vi "Logging Message Loop.vi"(8 "error in (no error)":errorcluster, 10 "Data Queue":refnum<queue>, 11 "Message Queues":T1) -> (0 "error out":errorcluster)   [LabVIEW 2019, in "Logging.lvlib"]
doc: "The message loop subVI to handle messages pertaining to logging data."
uses:
  Logging.lvlib
  support/Message Queue/All Message Queues.ctl
  support/Message Queue/Message Cluster.ctl
  Logging Configuration.ctl
  support/Message Queue/Message Queue.lvlib
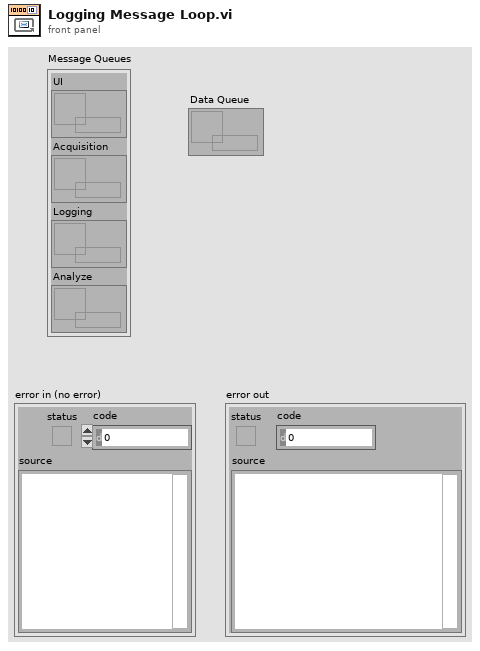
[diagram p1: front panel]
types:
  T1 = typedef "Message Queue.lvlib/All Message Queues.ctl" = cluster{"UI":refnum<queue>, "Acquisition":refnum<queue>, "Logging":refnum<queue>, "Analyze":refnum<queue>}
  T2 = typedef "Logging.lvlib/Logging Configuration.ctl" = cluster{"Log File Base Path":path, "Data Log Refnum":refnum<k1>}
  T3 = cluster{"Temperature Array":dbl[], "Average Range":dbl}
  T4 = enum16{"open", "replace", "create", "open or create", "replace or create", "replace or create with confirmation"}
  T5 = cluster{"Temperature Array":dbl[], "Average Range":dbl}[]
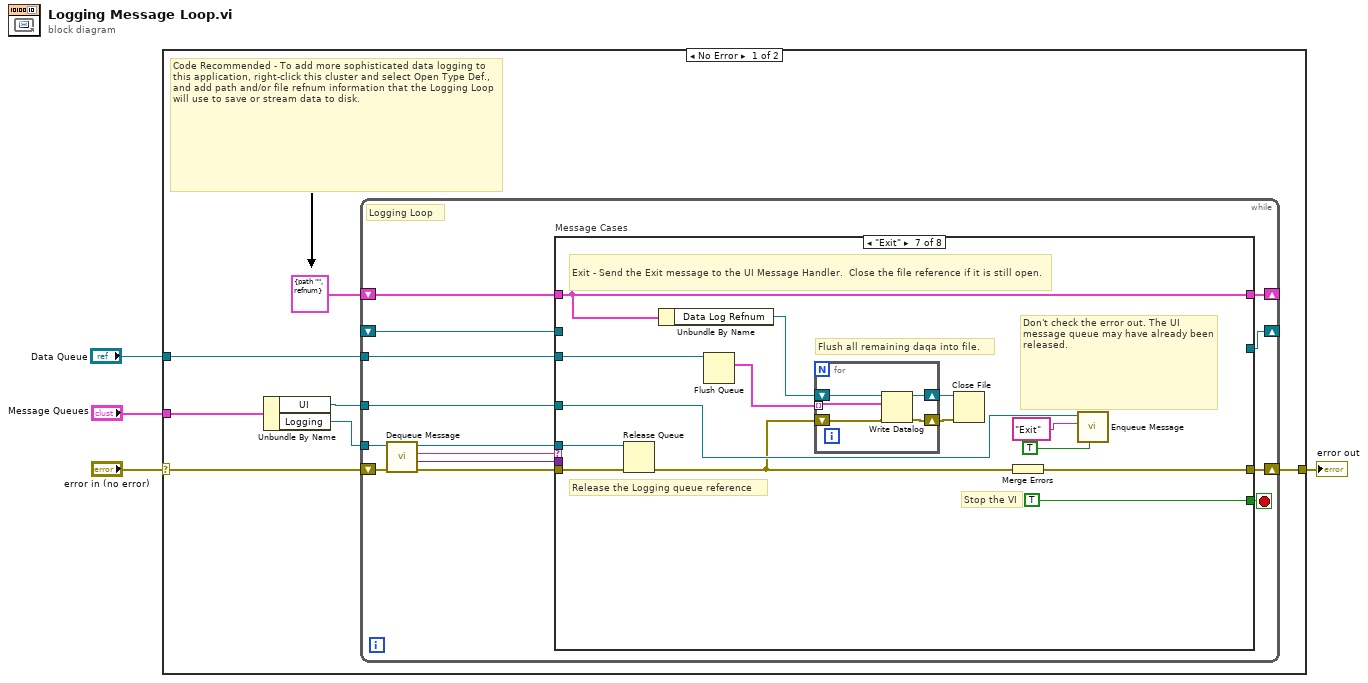
[diagram p0: block diagram]
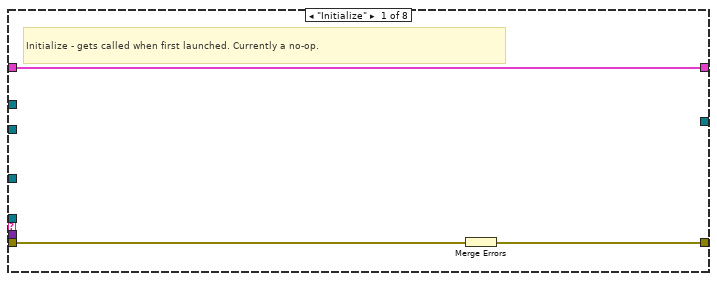
[diagram p2: hidden frame]
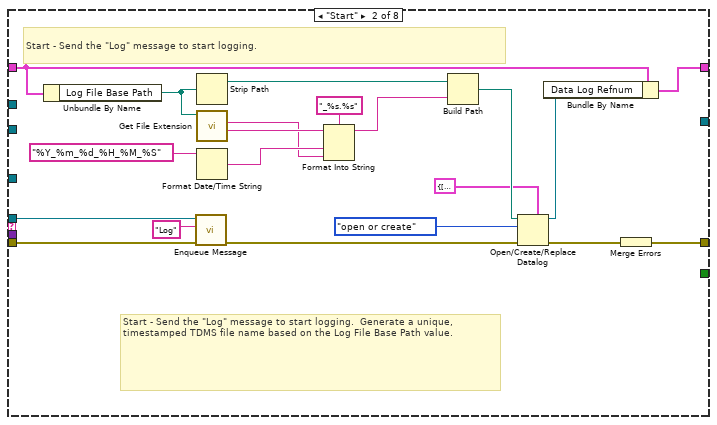
[diagram p3: hidden frame]
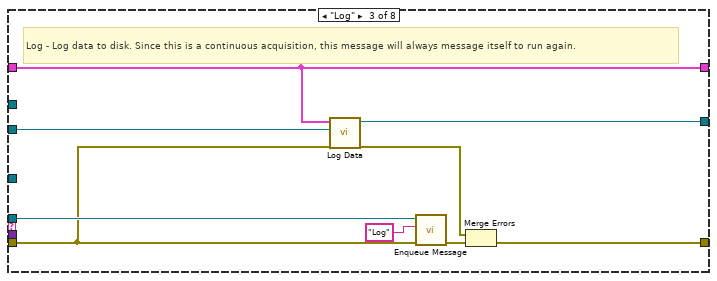
[diagram p4: hidden frame]
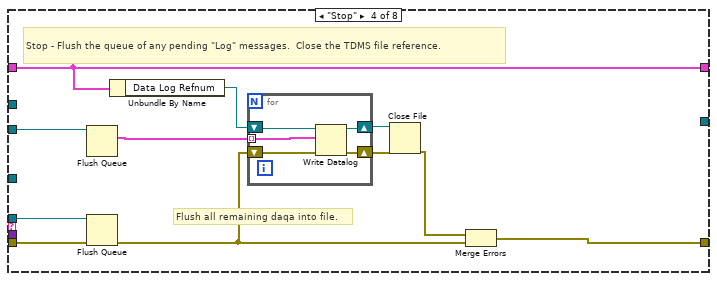
[diagram p5: hidden frame]
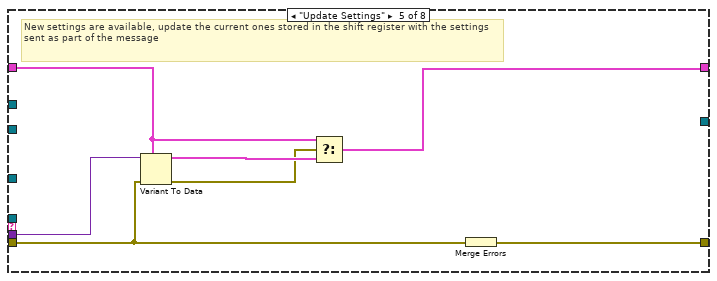
[diagram p6: hidden frame]
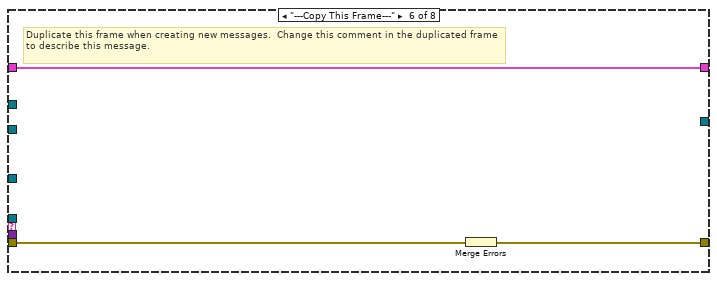
[diagram p7: hidden frame]
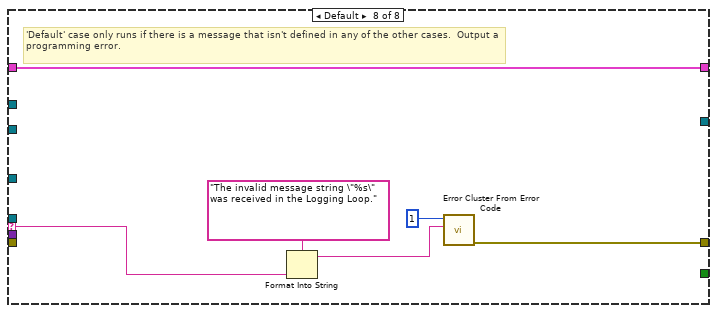
[diagram p8: hidden frame]
diagram:
  n1 = case shown="No Error" "error in (no error)" {
    selector: "error in (no error)" -> [w8 w109]
    tunnel: "Message Queues" -> [w11 _]
    tunnel: [w9 w109] -> w3
    tunnel: "Data Queue" -> [w7 _]
    frame No Error {
      # "Code Recommended - To add more sophisticated data logging to this application, right-click this cluster and select Open Type Def., and add path and/or file refnum information that the Logging Loop will use to save or stream data to disk."
      n2 = Unbundle By Name(w11) -> ("UI"=w6:refnum<queue>, "Logging"=w10:refnum<queue>)
      n3 = while {
        tunnel: w10 -> [w18]
        shift-right: [w24] -> w9
        shift-left: w8 -> [w23]
        tunnel: w6 -> [w17]
        tunnel: w7 -> [w16]
        shift-right: [w14] -> _
        shift-left: T2 {"Log File Base Path"=path "", "Data Log Refnum"=refnum} ("Logging Configuration") -> [w15]
        shift-right: [w13] -> _
        shift-left: _ -> [w12]
        stop <- w25 stop-if-true
        # "Logging Loop"
        n4 = call "Dequeue Message.vi"("error in (no error)"=w23, "Message Queue"=w18) -> ("error out"=w22:errorcluster, "Message Data"=w20:variant, "Message"=w21:string, "dup Message Queue"=w19:refnum<queue>)  [unwired: 6 in]
        n5 = case "Message Cases" shown="\"Exit\"" w21 {
          selector: w21 -> [_ _ _ _ _ _ _ w106]
          tunnel: w19 -> [_ w47 w55 w66 _ _ w91 _]
          tunnel: w22 -> [w26 w45 w53 w67 w74 w83 w94 _]
          tunnel: [w28 w48 w57 w68 w80 w81 w96 w104] -> w24
          tunnel: w15 -> [w27 w31 w51 w59 w78 w82 w90 w108]
          tunnel: [w27 w35 w51 w59 w75 w82 w90 w108] -> w14
          tunnel: [_ _ _ _ _ _ TRUE _] -> w25
          tunnel: w20 -> [_ _ _ _ w79 _ _ _]
          tunnel: w17 -> [_ _ _ _ _ _ w95 _]
          tunnel: w16 -> [_ _ w50 w63 _ _ w84 _]
          tunnel: [_ _ w49 _ _ _ _ _] -> w13
          tunnel: w12 -> [_ _ _ _ _ _ _ _]
          frame "Initialize" {
            # "Initialize - gets called when first launched. Currently a no-op."
            n6 = Merge Errors(w26) -> (w28:errorcluster)
          }
          frame "Start" {
            # "Start - Send the \"Log\" message to start logging."
            # "Start - Send the \"Log\" message to start logging.  Generate a unique, timestamped TDMS file name based on the Log File Base Path value."
            n7 = Unbundle By Name(w31) -> ("Log File Base Path"=w43:path)
            n8 = call "Enqueue Message.vi"("error in (no error)"=w45, "Message"="Log", "Message Queue"=w47) -> ("error out"=w34:errorcluster)  [unwired: 7 in, 1 out]
            n9 = Strip Path(path=w43) -> (stripped path=w42:path)  [unwired: 1 out]
            n10 = call <vilib>:"Get File Extension.vi"("file"=w43) -> ("filename without extension"=w41:string, "lowercase file extension"=w38:string)  [unwired: 6 in, 3 out]
            n11 = Format Date/Time String(time format string (%c)="%Y_%m_%d_%H_%M_%S") -> (date/time string=w39:string)  [unwired: 2 in]
            n12 = Format Into String(format string="_%s.%s", initial string=w41, w39, w38) -> (resulting string=w37:string)  [unwired: 1 in, 1 out]
            n13 = Build Path(base path=w42, name or relative path=w37) -> (appended path=w36:path)
            n14 = Open/Create/Replace Datalog(5:T3 {"Temperature Array"=[], "Average Range"=0.0} ("output cluster"), 8:w34, 10:T4."open or create" ("operation (0:open)"), 11:w36) -> (0:w33:errorcluster, 3:w29:refnum<k1>)  [unwired: 2 in, 1 out]
            n15 = Bundle By Name(cluster=w31, "Data Log Refnum"=w29) -> (w35:T2)
            n16 = Merge Errors(w33) -> (w48:errorcluster)
          }
          frame "Log" {
            # "Log - Log data to disk. Since this is a continuous acquisition, this message will always message itself to run again."
            n17 = call "Log Data.vi"("error in (no error)"=w53, "Data Queue"=w50, "Logging Configuration"=w51) -> ("error out"=w54:errorcluster, "Data Log Refnum"=w49:refnum<k1>)  [unwired: 7 in]
            n18 = call "Enqueue Message.vi"("error in (no error)"=w53, "Message"="Log", "Message Queue"=w55) -> ("error out"=w56:errorcluster)  [unwired: 7 in, 1 out]
            n19 = Merge Errors(w54, w56) -> (w57:errorcluster)
          }
          frame "Stop" {
            # "Flush all remaining daqa into file."
            # "Stop - Flush the queue of any pending \"Log\" messages.  Close the TDMS file reference."
            n20 = Flush Queue(queue=w63) -> (remaining elements=w58:T5)  [unwired: 1 in, 2 out]
            n21 = Flush Queue(queue=w66, error in (no error)=w67) -> (error out=w64:errorcluster)  [unwired: 2 out]
            n22 = Unbundle By Name(w59) -> ("Data Log Refnum"=w65:refnum<k1>)
            n23 = for {
              shift-right: [w70] -> w60
              shift-left: w65 -> [w71]
              shift-right: [w72] -> w62
              shift-left: w64 -> [w73]
              tunnel: w58 -> [w69] mode=indexing
              n24 = Write Datalog(4:w73, 6:w69, 7:w71) -> (0:w72:errorcluster, 3:w70:refnum<k1>)
            }
            n25 = Close File(refnum=w60, error in=w62) -> (error out=w61:errorcluster)  [unwired: 1 out]
            n26 = Merge Errors(w61, w64) -> (w68:errorcluster)
          }
          frame "Update Settings" {
            # "New settings are available, update the current ones stored in the shift register with the settings sent as part of the message"
            n27 = Variant To Data(error in=w74, type=w78, Variant=w79) -> (data=w77:T2, error out=w76:errorcluster)
            n28 = Select(t=w78, s=w76, f=w77) -> (s? t:f=w75:T2)
            n29 = Merge Errors(w74) -> (w80:errorcluster)
          }
          frame "---Copy This Frame---" {
            # "Duplicate this frame when creating new messages.  Change this comment in the duplicated frame to describe this message."
            n30 = Merge Errors(w83) -> (w81:errorcluster)
          }
          frame "Exit" {
            # "Flush all remaining daqa into file."
            # "Release the Logging queue reference"
            # "Don't check the error out. The UI message queue may have already been released."
            # "Stop the VI"
            # "Exit - Send the Exit message to the UI Message Handler.  Close the file reference if it is still open."
            n31 = Release Queue(queue=w91, error in (no error)=w94) -> (error out=w86:errorcluster)  [unwired: 1 in, 2 out]
            n32 = Unbundle By Name(w90) -> ("Data Log Refnum"=w85:refnum<k1>)
            n33 = Flush Queue(queue=w84) -> (remaining elements=w87:T5)  [unwired: 1 in, 2 out]
            n34 = for {
              tunnel: w87 -> [w98] mode=indexing
              shift-right: [w100] -> w88
              shift-left: w85 -> [w99]
              shift-right: [w101] -> w89
              shift-left: w86 -> [w102]
              n35 = Write Datalog(4:w102, 6:w98, 7:w99) -> (0:w101:errorcluster, 3:w100:refnum<k1>)
            }
            n36 = Close File(refnum=w88, error in=w89) -> ()  [unwired: 2 out]
            n37 = Merge Errors(w86) -> (w96:errorcluster)
            n38 = call "Enqueue Message.vi"("Priority Message? (F)"=TRUE, "Message"="Exit", "Message Queue"=w95) -> ()  [unwired: 7 in, 2 out]
          }
          frame Default {
            # "'Default' case only runs if there is a message that isn't defined in any of the other cases.  Output a programming error."
            n39 = Format Into String(format string="The invalid message string \"%s\" was received in the Logging Loop." ("Invalid Logging Message"), w106) -> (resulting string=w103:string)  [unwired: 2 in, 1 out]
            n40 = call <vilib>:"Error Cluster From Error Code.vi"("error message (\"\")"=w103, "error code (0)"=1) -> ("error out"=w104:errorcluster)  [unwired: 7 in]
          }
        }
      }
    }
    frame Error {
    }
  }
  "error out" <- w3
